vi "GetNumFromName.vi"(10 "name":string, 11 "dvotAFTKinetics":refnum<class "dvotAFTKinetics.lvclass">) -> (2 "Numeric":i32, 3 "dvotAFTKinetics":refnum<class "dvotAFTKinetics.lvclass">)   [LabVIEW 2012, in "dvotAFTKinetics.lvclass"]
uses:
  dvotAFTKinetics.lvclass
  Constants/dvotAFTConstants.vi
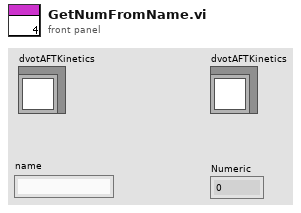
[diagram p1: front panel]
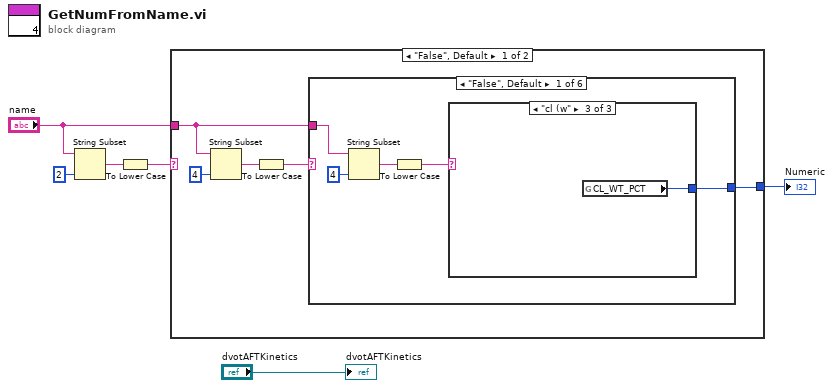
[diagram p0: block diagram]
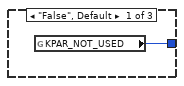
[diagram p2: hidden frame]
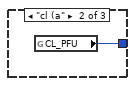
[diagram p3: hidden frame]
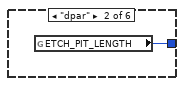
[diagram p4: hidden frame]
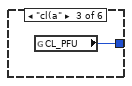
[diagram p5: hidden frame]
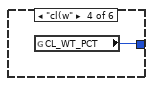
[diagram p6: hidden frame]
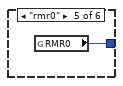
[diagram p7: hidden frame]
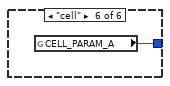
[diagram p8: hidden frame]
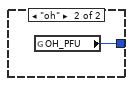
[diagram p9: hidden frame]
diagram:
  n1 = String Subset(string="name", length (rest)=2 ("length (rest)")) -> (substring=w6:string)  [unwired: 1 in]
  n2 = To Lower Case(string=w6) -> (all lower case string=w4:string)
  n3 = case shown="\"False\", Default" w4 {
    tunnel: "name" -> [w7 _]
    tunnel: [w8 w25] -> w2
    frame "False", Default {
      n4 = String Subset(string=w7, length (rest)=4 ("length (rest)")) -> (substring=w11:string)  [unwired: 1 in]
      n5 = To Lower Case(string=w11) -> (all lower case string=w9:string)
      n6 = case shown="\"False\", Default" w9 {
        tunnel: [w16 w20 w21 w22 w23 w24] -> w8
        tunnel: w7 -> [w13 _ _ _ _ _]
        frame "False", Default {
          n7 = String Subset(string=w13, length (rest)=4 ("length (rest)")) -> (substring=w15:string)  [unwired: 1 in]
          n8 = To Lower Case(string=w15) -> (all lower case string=w12:string)
          n9 = case shown="\"cl (w\"" w12 {
            tunnel: [w17 w18 w19] -> w16
            frame "False", Default {
              n10 = global read "dvotAFTConstants.vi" "KPAR_NOT_USED"() -> (w17:i32)
            }
            frame "cl (a" {
              n11 = global read "dvotAFTConstants.vi" "CL_PFU"() -> (w18:i32)
            }
            frame "cl (w" {
              n12 = global read "dvotAFTConstants.vi" "CL_WT_PCT"() -> (w19:i32)
            }
          }
        }
        frame "dpar" {
          n13 = global read "dvotAFTConstants.vi" "ETCH_PIT_LENGTH"() -> (w20:i32)
        }
        frame "cl(a" {
          n14 = global read "dvotAFTConstants.vi" "CL_PFU"() -> (w21:i32)
        }
        frame "cl(w" {
          n15 = global read "dvotAFTConstants.vi" "CL_WT_PCT"() -> (w22:i32)
        }
        frame "rmr0" {
          n16 = global read "dvotAFTConstants.vi" "RMR0"() -> (w23:i32)
        }
        frame "cell" {
          n17 = global read "dvotAFTConstants.vi" "CELL_PARAM_A"() -> (w24:i32)
        }
      }
    }
    frame "oh" {
      n18 = global read "dvotAFTConstants.vi" "OH_PFU"() -> (w25:i32)
    }
  }
  "Numeric" <- w2
  "dvotAFTKinetics" <- "dvotAFTKinetics"
